vi "StartRecord.vi"(8 "error in (no error)":errorcluster, 10 "Label":string, 11 "Task_Abstr in":refnum<class "Task_Abstr.lvclass">) -> (0 "error out":errorcluster, 3 "Task_Abstr out":refnum<class "Task_Abstr.lvclass">)   [LabVIEW 2025, in "Task_Abstr.lvlib" / "Task_Abstr.lvclass"]
uses:
  Task_Abstr.lvclass
  WaveformData.ctl
  <vilib>/Utility/miscctls.llb/LVMapReplaceAction.ctl
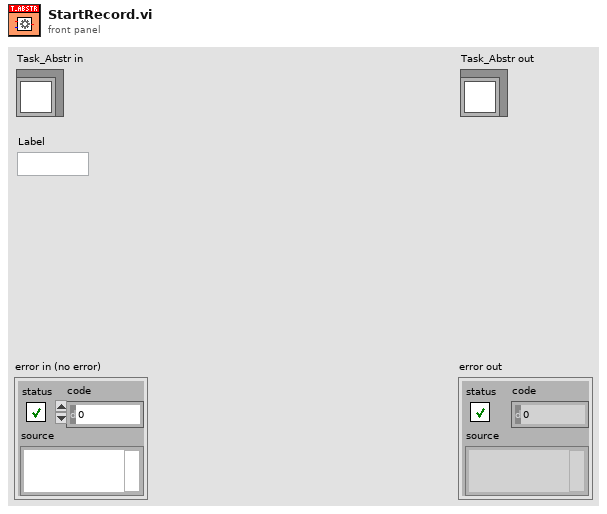
[diagram p1: front panel]
types:
  T1 = typedef "Task_Abstr.lvlib/Task_Abstr.lvclass/WaveformData.ctl" = cluster{"StartTime":timestamp, "StopTime":timestamp, "Waveform":waveform(dbl)[]}
  T2 = typedef "LVMapReplaceAction.ctl" = enum32{"Modify Entry only if found", "Add or Modify Entry", "Delete Entry"}
  T3 = typedef "Task_Abstr.lvlib/Task_Abstr.lvclass/DataContainer.ctl" = map{string, T1}
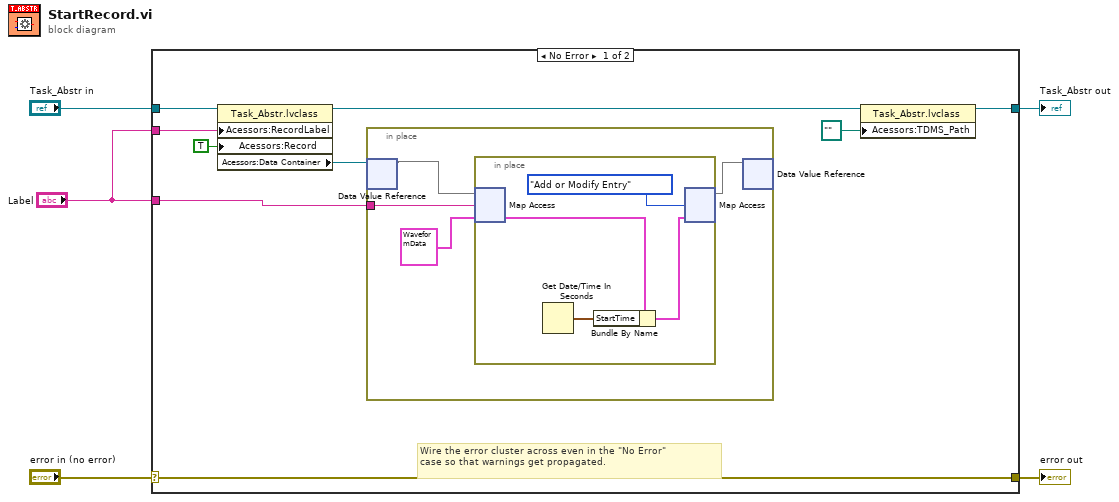
[diagram p0: block diagram]
diagram:
  n1 = case shown="No Error" "error in (no error)" {
    selector: "error in (no error)" -> [w14 w24]
    tunnel: [w14 w24] -> w4
    tunnel: [w8 w23] -> w2
    tunnel: "Task_Abstr in" -> [w13 w23]
    tunnel: "Label" -> [w11 _]
    tunnel: "Label" -> [w9 _]
    frame No Error {
      # "Wire the error cluster across even in the \"No Error\"\ncase so that warnings get propagated."
      n2 = property class="Task_Abstr.lvclass"(reference=w13, "Acessors:RecordLabel"=w11, "Acessors:Record"=TRUE ("Record")) -> (reference out=w12:refnum<class "Task_Abstr.lvclass">, "Acessors:Data Container"=w6:refnum<data-value>)  [unwired: 1 in, 1 out]
      n3 = in-place {
        in-place-border: w9 -> [w18]
        n4 = in-place-dvr #1(w6) -> (w16:T3)  [unwired: 1 out]
        n5 = in-place {
          n6 = in-place-map #2(w16, w18, T1 {"StartTime"=timestamp(0 s since 1904-01-01), "StopTime"=timestamp(0 s since 1904-01-01), "Waveform"=[]} ("WaveformData")) -> (w19:T1)  [unwired: 1 out]
          n7 = Get Date/Time In Seconds() -> (seconds since 1Jan1904=w20:timestamp)
          n8 = Bundle By Name(cluster=w19, "StartTime"=w20) -> (w21:T1)
          n9 = in-place-map #2(w21, LVMapReplaceAction."Add or Modify Entry" ("action")) -> (w15:T3)  [unwired: 2 out]
        }
        n10 = in-place-dvr #1(w15) -> ()  [unwired: 2 out]
      }
      n11 = property class="Task_Abstr.lvclass"(reference=w12, "Acessors:TDMS_Path"=path "" ("TDMS_Path")) -> (reference out=w8:refnum<class "Task_Abstr.lvclass">)  [unwired: 1 in, 1 out]
    }
    frame Error {
    }
  }
  "error out" <- w4
  "Task_Abstr out" <- w2
